vi "PixelToScanCoordinateConvFactors.vi"(6 "Header":T2, 9 "Scan Plane":i32, 11 "Coordinate Data":dbl[][][][](array[numeric])) -> (3 "PixelToScanCoordConvFactors":T1 {"Dz_dcol" format="%0.2f"; "Dy_dcol" format="%0.2f"; "Dx_dcol" format="%0.2f"; "Dz_drow" format="%0.2f"; "Dy_drow" format="%0.2f"; "Dx_drow" format="%0.2f"})   [LabVIEW 2012]
uses:
  <vilib>/Analysis/NI_AALPro.lvlib
  <vilib>/Analysis/NI_AALBase.lvlib
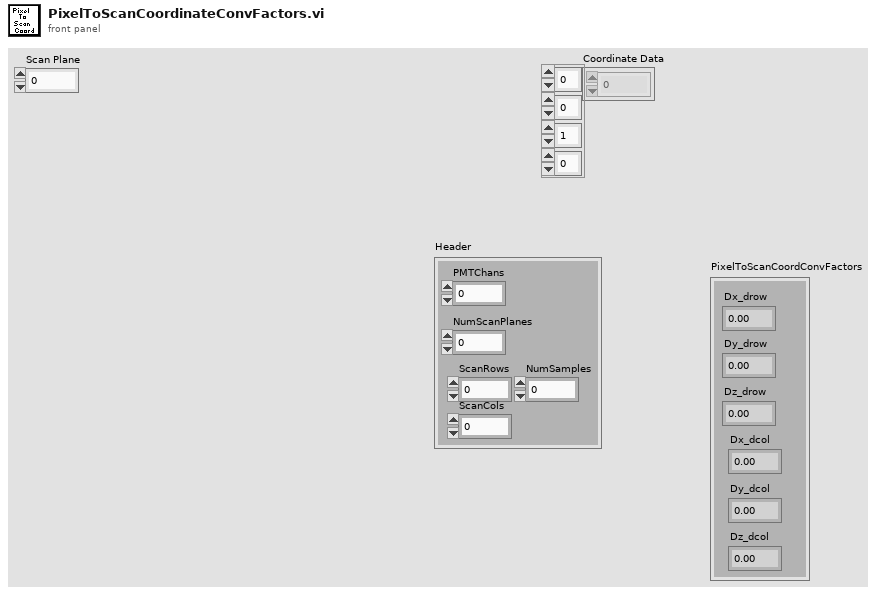
[diagram p1: front panel]
types:
  T1 = cluster{"Dx_drow":dbl, "Dy_drow":dbl, "Dz_drow":dbl, "Dx_dcol":dbl, "Dy_dcol":dbl, "Dz_dcol":dbl}
  T2 = cluster{"PMTChans":i32, "NumScanPlanes":i32, "ScanRows":i32, "ScanCols":i32, "NumSamples":i32}
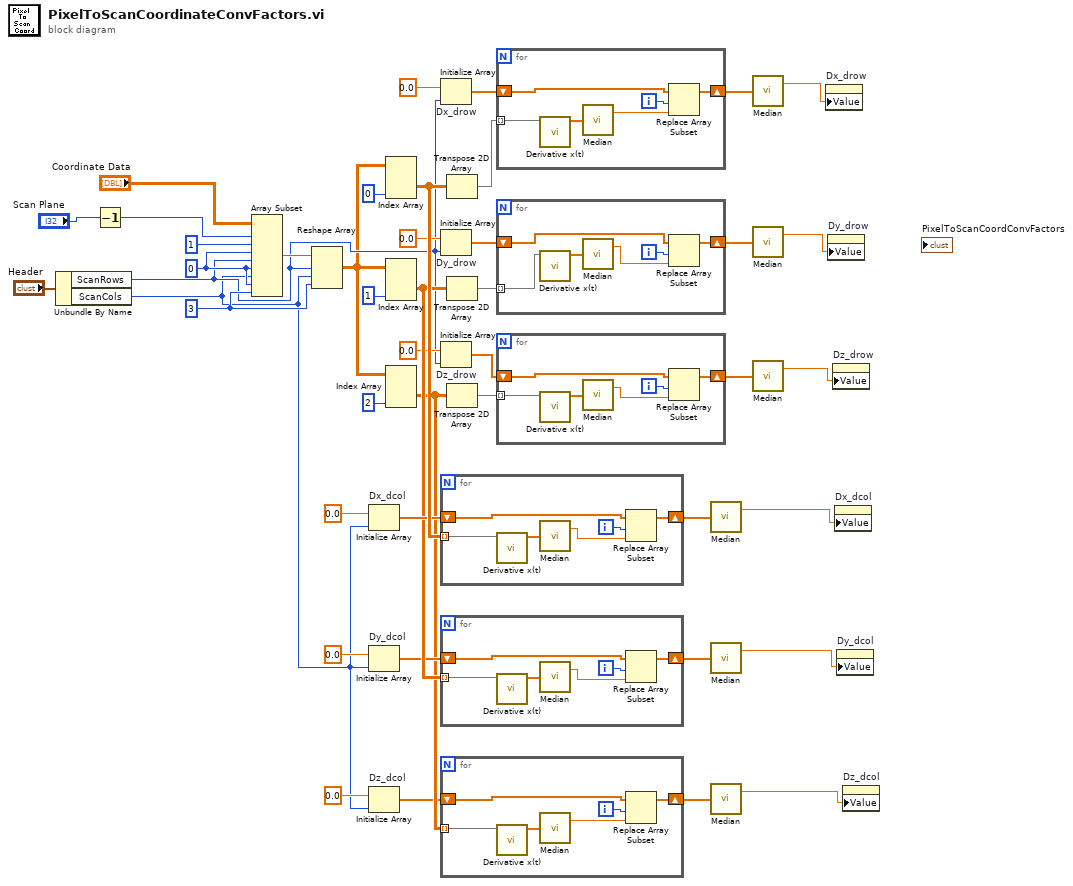
[diagram p0: block diagram]
diagram:
  w39 = 3 ("length")
  w41 = 0 ("index")
  n1 = Unbundle By Name("Header") -> ("ScanRows"=w17:i32, "ScanCols"=w16:i32)
  n2 = Decrement(x="Scan Plane") -> (x-1=w1:i32)
  n3 = Array Subset(array="Coordinate Data", index (dim 0)=w1, length (dim 0)=1 ("length"), index (dim 1)=w41, length (dim 1)=w17, index (dim 2)=w41, length (dim 2)=w16, index (dim 3)=w41, length (dim 3)=w39) -> (w40:dbl[][][][])
  n4 = Reshape Array(w40, w17, w16, w39) -> (w15:dbl[][][])
  n5 = Initialize Array "Dx_dcol"(0.0 ("element"), w16) -> (w35:dbl[])
  n6 = Initialize Array "Dy_dcol"(0.0 ("element"), w16) -> (w28:dbl[])
  n7 = Initialize Array "Dz_dcol"(0.0 ("element"), w16) -> (w21:dbl[])
  n8 = Index Array(array=w15, index (dim 2)=0 ("disabled index (col)")) -> (element=w37:dbl[][])  [unwired: 2 in]
  n9 = Index Array(array=w15, index (dim 2)=1 ("disabled index (col)")) -> (element=w30:dbl[][])  [unwired: 2 in]
  n10 = Index Array(array=w15, index (dim 2)=2 ("disabled index (col)")) -> (element=w23:dbl[][])  [unwired: 2 in]
  n11 = Initialize Array "Dx_drow"(0.0 ("element"), w17) -> (w33:dbl[])
  n12 = Initialize Array "Dy_drow"(0.0 ("element"), w17) -> (w26:dbl[])
  n13 = Initialize Array "Dz_drow"(0.0 ("element"), w17) -> (w19:dbl[])
  n14 = for {
    tunnel: w37 -> [w50] mode=indexing
    shift-right: [w48] -> w9
    shift-left: w35 -> [w49]
    i -> [w47]
    n15 = call <vilib>:"Derivative x(t).vi"("X"=w50) -> ("dX/dt"=w45:dbl[])  [unwired: 9 in, 1 out]
    n16 = call <vilib>:"Median.vi"("X"=w45) -> ("median"=w46:dbl)  [unwired: 1 out]
    n17 = Replace Array Subset(array=w49, new element=w46, index=w47) -> (w48:dbl[])
  }
  n18 = for {
    tunnel: w30 -> [w56] mode=indexing
    shift-right: [w54] -> w10
    shift-left: w28 -> [w55]
    i -> [w53]
    n19 = call <vilib>:"Derivative x(t).vi"("X"=w56) -> ("dX/dt"=w52:dbl[])  [unwired: 9 in, 1 out]
    n20 = call <vilib>:"Median.vi"("X"=w52) -> ("median"=w51:dbl)  [unwired: 1 out]
    n21 = Replace Array Subset(array=w55, new element=w51, index=w53) -> (w54:dbl[])
  }
  n22 = for {
    tunnel: w23 -> [w62] mode=indexing
    shift-right: [w60] -> w13
    shift-left: w21 -> [w61]
    i -> [w59]
    n23 = call <vilib>:"Derivative x(t).vi"("X"=w62) -> ("dX/dt"=w58:dbl[])  [unwired: 9 in, 1 out]
    n24 = call <vilib>:"Median.vi"("X"=w58) -> ("median"=w57:dbl)  [unwired: 1 out]
    n25 = Replace Array Subset(array=w61, new element=w57, index=w59) -> (w60:dbl[])
  }
  n26 = Transpose 2D Array(2D array=w37) -> (transposed array=w34:dbl[][])
  n27 = Transpose 2D Array(2D array=w30) -> (transposed array=w27:dbl[][])
  n28 = Transpose 2D Array(2D array=w23) -> (transposed array=w20:dbl[][])
  n29 = for {
    tunnel: w34 -> [w68] mode=indexing
    shift-right: [w66] -> w14
    shift-left: w33 -> [w67]
    i -> [w65]
    n30 = call <vilib>:"Derivative x(t).vi"("X"=w68) -> ("dX/dt"=w64:dbl[])  [unwired: 9 in, 1 out]
    n31 = call <vilib>:"Median.vi"("X"=w64) -> ("median"=w63:dbl)  [unwired: 1 out]
    n32 = Replace Array Subset(array=w67, new element=w63, index=w65) -> (w66:dbl[])
  }
  n33 = for {
    tunnel: w27 -> [w74] mode=indexing
    shift-right: [w72] -> w12
    shift-left: w26 -> [w73]
    i -> [w71]
    n34 = call <vilib>:"Derivative x(t).vi"("X"=w74) -> ("dX/dt"=w70:dbl[])  [unwired: 9 in, 1 out]
    n35 = call <vilib>:"Median.vi"("X"=w70) -> ("median"=w69:dbl)  [unwired: 1 out]
    n36 = Replace Array Subset(array=w73, new element=w69, index=w71) -> (w72:dbl[])
  }
  n37 = for {
    tunnel: w20 -> [w80] mode=indexing
    shift-right: [w78] -> w11
    shift-left: w19 -> [w79]
    i -> [w77]
    n38 = call <vilib>:"Derivative x(t).vi"("X"=w80) -> ("dX/dt"=w76:dbl[])  [unwired: 9 in, 1 out]
    n39 = call <vilib>:"Median.vi"("X"=w76) -> ("median"=w75:dbl)  [unwired: 1 out]
    n40 = Replace Array Subset(array=w79, new element=w75, index=w77) -> (w78:dbl[])
  }
  n41 = call <vilib>:"Median.vi"("X"=w9) -> ("median"=w5:dbl)  [unwired: 1 out]
  n42 = call <vilib>:"Median.vi"("X"=w10) -> ("median"=w4:dbl)  [unwired: 1 out]
  n43 = call <vilib>:"Median.vi"("X"=w13) -> ("median"=w3:dbl)  [unwired: 1 out]
  n44 = call <vilib>:"Median.vi"("X"=w14) -> ("median"=w8:dbl)  [unwired: 1 out]
  n45 = call <vilib>:"Median.vi"("X"=w12) -> ("median"=w7:dbl)  [unwired: 1 out]
  n46 = call <vilib>:"Median.vi"("X"=w11) -> ("median"=w6:dbl)  [unwired: 1 out]
  n47 = property on="Dx_drow" class="DigNum (strict)"("Value"=w8) -> ()  [unwired: 2 in, 2 out]
  n48 = property on="Dy_drow" class="DigNum (strict)"("Value"=w7) -> ()  [unwired: 2 in, 2 out]
  n49 = property on="Dz_drow" class="DigNum (strict)"("Value"=w6) -> ()  [unwired: 2 in, 2 out]
  n50 = property on="Dx_dcol" class="DigNum (strict)"("Value"=w5) -> ()  [unwired: 2 in, 2 out]
  n51 = property on="Dy_dcol" class="DigNum (strict)"("Value"=w4) -> ()  [unwired: 2 in, 2 out]
  n52 = property on="Dz_dcol" class="DigNum (strict)"("Value"=w3) -> ()  [unwired: 2 in, 2 out]
